vi "Close Instrument.vi"(8 "error in (no error)":errorcluster, 11 "Simulated DMM.lvclass in":refnum<class "Simulated DMM.lvclass">) -> (0 "error out":errorcluster, 3 "Simulated DMM.lvclass out":refnum<class "Simulated DMM.lvclass">)   [LabVIEW 2010, in "Simulated DMM.lvclass"]
uses:
  Simulated DMM.lvclass
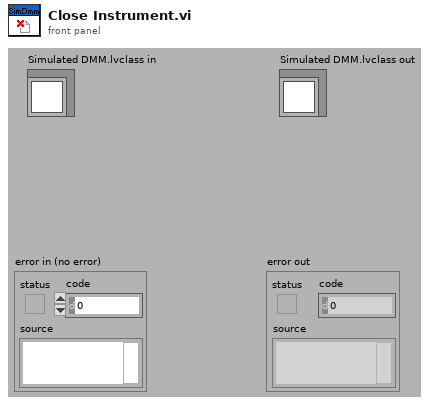
[diagram p1: front panel]
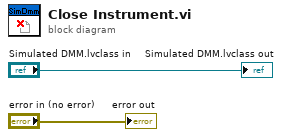
[diagram p0: block diagram]
diagram:
  "error out" <- "error in (no error)"
  "Simulated DMM.lvclass out" <- "Simulated DMM.lvclass in"
